vi "Frame1.vi"() -> ()   [LabVIEW 2017]
uses:
  <vilib>/myRIO/Instrument Drivers/Onboard IO/DIO/typedefs/DIO Reference.ctl
  <vilib>/myRIO/Common/Instrument Driver Framework/Utilities/typedefs/myRIO Generic Hardware Reference.ctl
  <vilib>/myRIO/Common/Instrument Driver Framework/Utilities/typedefs/Hardware Version Enum.ctl
  <vilib>/myRIO/Common/Instrument Driver Framework/Utilities/typedefs/myRIO v1.0 Reference.ctl
  <vilib>/myRIO/Common/Instrument Driver Framework/Utilities/typedefs/Generic FPGA Reference.ctl
  <vilib>/myRIO/Common/Instrument Driver Framework/myRIO v1.0/DIO/typedefs/DIO Channels List.ctl
  <vilib>/myRIO/Common/Instrument Driver Framework/myRIO v1.0/DIO/typedefs/DIO Channels Enum.ctl
  <vilib>/userdefined/High Color/nirio_resource_hc.ctl
  <vilib>/myRIO/Common/Instrument Driver Framework/Utilities/vis/Is FPGA Ref Available.vi
  <vilib>/myRIO/Common/Instrument Driver Framework/myRIO v1.0/DIO/vis/myRIO v1.1 Open DIO.vi
  <vilib>/myRIO/Instrument Drivers/Onboard IO/DIO/vis/Read.vi
  <vilib>/myRIO/Common/Instrument Driver Framework/Utilities/vis/Validate Channels.vi
  <vilib>/myRIO/Common/Instrument Driver Framework/myRIO v1.0/DIO/vis/myRIO v1.0 Reserve DIO.vi
  <vilib>/myRIO/Common/Instrument Driver Framework/myRIO v1.0/UART/vis/myRIO v1.0 Close UART.vi
  <vilib>/myRIO/Common/Instrument Driver Framework/myRIO v1.0/Resource Manager/vis/myRIO v1.0 Reserve Channel List.vi
  <vilib>/myRIO/Common/Instrument Driver Framework/myRIO v1.0/DIO/vis/myRIO v1.0 Build MUX Configuration DIO.vi
  <vilib>/myRIO/Common/Instrument Driver Framework/myRIO v1.0/Resource Manager/vis/myRIO v1.0 Reserve Channel.vi
  <vilib>/myRIO/Common/Instrument Driver Framework/myRIO v1.0/Resource Manager/vis/myRIO v1.0 Unreserve Channel.vi
  <vilib>/myRIO/Common/Instrument Driver Framework/myRIO v1.0/Resource Manager/vis/myRIO v1.0 Create Configuration List.vi
  <vilib>/myRIO/Common/Instrument Driver Framework/myRIO v1.0/Resource Manager/vis/myRIO v1.0 Build Mutex Name.vi
  <vilib>/Utility/VariantDataType/GetNumericInfo.vi
  <vilib>/Utility/error.llb/Error Cluster From Error Code.vi
  <vilib>/myRIO/Common/Instrument Driver Framework/myRIO v1.0/myRIO v1.1 Open.vi
  <vilib>/myRIO/Common/Instrument Driver Framework/Utilities/vis/IO Manager.vi
  <vilib>/myRIO/Common/Instrument Driver Framework/Utilities/vis/Configuration Manager.vi
  <vilib>/myRIO/Common/Instrument Driver Framework/myRIO v1.0/Resource Manager/vis/myRIO v1.0 Configure IO.vi
  <vilib>/myRIO/Common/Instrument Driver Framework/myRIO v1.0/myRIO v1.0 Close.vi
  <vilib>/myRIO/Common/Instrument Driver Framework/myRIO v1.0/DIO/vis/myRIO v1.0 Read DIO.vi
  <vilib>/myRIO/Common/Instrument Driver Framework/Utilities/vis/FPGA Ref Manager.vi
  <vilib>/myRIO/Common/Instrument Driver Framework/myRIO v1.0/myRIO v1.0 Reset FPGA.vi
  <vilib>/myRIO/Common/Instrument Driver Framework/myRIO v1.0/IRQ/vis/myRIO v1.0 IRQ Info FGV.vi
  <vilib>/myRIO/Common/Instrument Driver Framework/myRIO v1.0/IRQ/vis/myRIO v1.0 Timer IRQ Info FGV.vi
  <vilib>/myRIO/Common/Instrument Driver Framework/myRIO v1.0/IRQ/vis/myRIO v1.0 ISR Agent.vi
  <vilib>/myRIO/Express VI/Onboard Devices/Button/Button Express VI.xnode
  <vilib>/myRIO/Instrument Drivers/Onboard IO/DIO/vis/myRIO DIO Open.xnode
  <vilib>/myRIO/Instrument Drivers/Onboard IO/DIO/DIO.lvlib
  <vilib>/myRIO/Instrument Drivers/Utilities/Utilities.lvlib
panel:
  out "error out":errorcluster
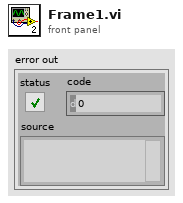
[diagram p1: front panel]
types:
  T1 = typedef "DIO.lvlib/DIO Reference.ctl" = cluster{"myRIO Reference":T2, "DIO Channels List":T6}
  T2 = typedef "myRIO Generic Hardware Reference.ctl" = cluster{"myRIO Model":T3, "myRIO Hardware Reference":T4}
  T3 = typedef "Hardware Version Enum.ctl" = enum16{"Unknown", "myRIO-1900", "myRIO-1950", "roboRIO", "NI ELVIS RIO CM"}
  T4 = typedef "myRIO v1.0 Reference.ctl" = cluster{"Generic FPGA Reference":T5, "Allow multiple opens":bool}
  T5 = typedef "Generic FPGA Reference.ctl" = refnum<k20>
  T6 = typedef "DIO Channels List.ctl" = T7[]
  T7 = typedef "DIO Channels Enum.ctl" = enum16{"Not Connected", "C/DIO0", "C/DIO1", "C/DIO2", "C/DIO3", "C/DIO4", "C/DIO5", "C/DIO6", "C/DIO7", "A/DIO0", "A/DIO1", "A/DIO2", "A/DIO3", "A/DIO4", "A/DIO5", "A/DIO6", "A/DIO7", "A/DIO8", "A/DIO9", "A/DIO10", "A/DIO11", "A/DIO12", "A/DIO13", "A/DIO14", "A/DIO15", "B/DIO0", "B/DIO1", "B/DIO2", "B/DIO3", "B/DIO4", "B/DIO5", "B/DIO6", "B/DIO7", "B/DIO8", "B/DIO9", "B/DIO10", "B/DIO11", "B/DIO12", "B/DIO13", "B/DIO14", "B/DIO15", "LED0", "LED1", "LED2", "LED3", "Button0", "DIO/DIO0", "DIO/DIO1", "DIO/DIO2", "DIO/DIO3", "DIO/DIO4", "DIO/DIO5", "DIO/DIO6", "DIO/DIO7", "DIO/DIO8", "DIO/DIO9", "SPI/CS0", "SPI/CS1", "SPI/CS2", "SPI/CS3", "LED RADIO (Green)", "LED RADIO (Red)", "LED COMM (Green)", "LED COMM (Red)", "LED MODE (Green)", "LED MODE (Red)"}
  T8 = typedef "nirio_resource_hc.ctl" = tag
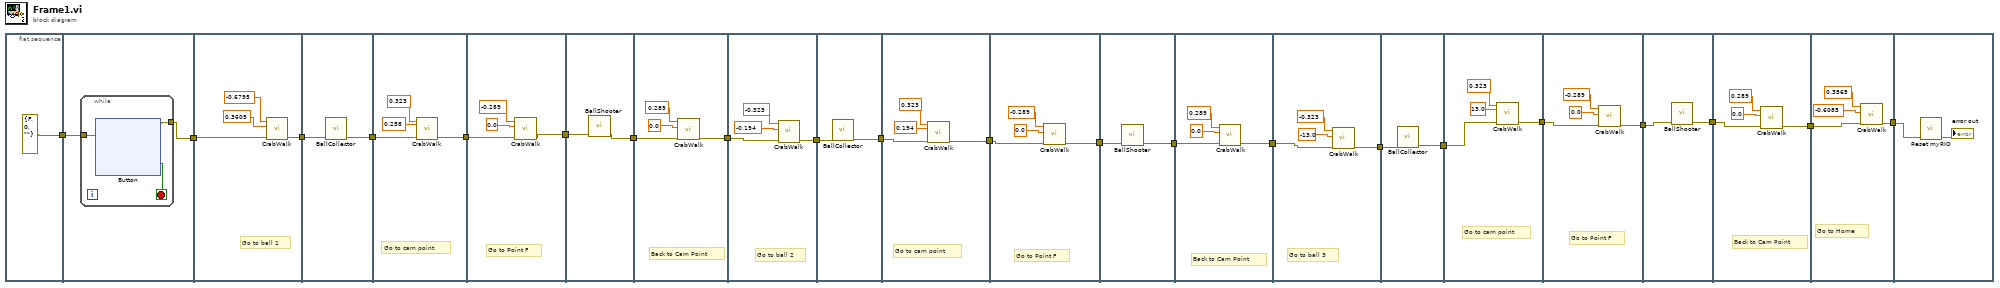
[diagram p0: block diagram]
diagram:
  n1 = flat-sequence {
    tunnel: [errorcluster {"status"=FALSE, "code"=0, "source"=""} ("error constant")] -> w21
    tunnel: w21 -> [w24]
    tunnel: [w23] -> w20
    tunnel: w20 -> [w66]
    tunnel: [w65] -> w19
    tunnel: w19 -> [w68]
    tunnel: [w67] -> w18
    tunnel: w18 -> [w72]
    tunnel: [w71] -> w17
    tunnel: w17 -> [w76]
    tunnel: [w73] -> w16
    tunnel: w16 -> [w78]
    tunnel: [w77] -> w15
    tunnel: w15 -> [w80]
    tunnel: [w79] -> w14
    tunnel: w14 -> [w84]
    tunnel: [w83] -> w13
    tunnel: w13 -> [w88]
    tunnel: [w87] -> w12
    tunnel: w12 -> [w90]
    tunnel: [w89] -> w11
    tunnel: w11 -> [w94]
    tunnel: [w93] -> w10
    tunnel: w10 -> [w98]
    tunnel: [w97] -> w9
    tunnel: w9 -> [w100]
    tunnel: [w99] -> w8
    tunnel: w8 -> [w104]
    tunnel: [w103] -> w7
    tunnel: w7 -> [w108]
    tunnel: [w107] -> w6
    tunnel: w6 -> [w110]
    tunnel: [w109] -> w5
    tunnel: w5 -> [w114]
    tunnel: [w113] -> w4
    tunnel: w4 -> [w118]
    tunnel: [w117] -> w3
    tunnel: w3 -> [w120]
    tunnel: [w119] -> w2
    tunnel: w2 -> [w124]
    tunnel: [w123] -> w1
    tunnel: w1 -> [w127]
    frame #0 {
    }
    frame #1 {
      n2 = while {
        tunnel: w24 -> [w27]
        tunnel: [w25] -> w23
        stop <- w26 stop-if-true
        n3 = xnode "Button"("error in (no error)"=w27) -> ("Value"=w26:bool, "error out"=w25:errorcluster)
      }
    }
    frame #2 {
      # "Go to ball 1"
      n4 = call "CrabWalk.vi"("error in\n(no error)"=w66, "Distance Y (m)"=0.3605, "Distance X (m)"=-0.6795) -> ("error out"=w65:errorcluster)  [unwired: 7 in, 1 out]
    }
    frame #3 {
      n5 = call "BallCollector.vi"("error in\n(no error)"=w68) -> ("error out"=w67:errorcluster)  [unwired: 10 in]
    }
    frame #4 {
      # "Go to cam point"
      n6 = call "CrabWalk.vi"("error in\n(no error)"=w72, "Distance Y (m)"=0.258, "Distance X (m)"=0.323) -> ("error out"=w71:errorcluster)  [unwired: 7 in, 1 out]
    }
    frame #5 {
      # "Go to Point F"
      n7 = call "CrabWalk.vi"("error in\n(no error)"=w76, "Distance Y (m)"=0.0, "Distance X (m)"=-0.289) -> ("error out"=w73:errorcluster)  [unwired: 7 in, 1 out]
    }
    frame #6 {
      n8 = call "BallShooter.vi"("error in (no error)"=w78) -> ("error out"=w77:errorcluster)  [unwired: 10 in]
    }
    frame #7 {
      # "Back to Cam Point"
      n9 = call "CrabWalk.vi"("error in\n(no error)"=w80, "Distance Y (m)"=0.0, "Distance X (m)"=0.289) -> ("error out"=w79:errorcluster)  [unwired: 7 in, 1 out]
    }
    frame #8 {
      # "Go to ball 2"
      n10 = call "CrabWalk.vi"("error in\n(no error)"=w84, "Distance Y (m)"=-0.194, "Distance X (m)"=-0.323) -> ("error out"=w83:errorcluster)  [unwired: 7 in, 1 out]
    }
    frame #9 {
      n11 = call "BallCollector.vi"("error in\n(no error)"=w88) -> ("error out"=w87:errorcluster)  [unwired: 10 in]
    }
    frame #10 {
      # "Go to cam point"
      n12 = call "CrabWalk.vi"("error in\n(no error)"=w90, "Distance Y (m)"=0.194, "Distance X (m)"=0.323) -> ("error out"=w89:errorcluster)  [unwired: 7 in, 1 out]
    }
    frame #11 {
      # "Go to Point F"
      n13 = call "CrabWalk.vi"("error in\n(no error)"=w94, "Distance Y (m)"=0.0, "Distance X (m)"=-0.289) -> ("error out"=w93:errorcluster)  [unwired: 7 in, 1 out]
    }
    frame #12 {
      n14 = call "BallShooter.vi"("error in (no error)"=w98) -> ("error out"=w97:errorcluster)  [unwired: 10 in]
    }
    frame #13 {
      # "Back to Cam Point"
      n15 = call "CrabWalk.vi"("error in\n(no error)"=w100, "Distance Y (m)"=0.0, "Distance X (m)"=0.289) -> ("error out"=w99:errorcluster)  [unwired: 7 in, 1 out]
    }
    frame #14 {
      # "Go to ball 3"
      n16 = call "CrabWalk.vi"("error in\n(no error)"=w104, "Distance Y (m)"=-13.0, "Distance X (m)"=-0.323) -> ("error out"=w103:errorcluster)  [unwired: 7 in, 1 out]
    }
    frame #15 {
      n17 = call "BallCollector.vi"("error in\n(no error)"=w108) -> ("error out"=w107:errorcluster)  [unwired: 10 in]
    }
    frame #16 {
      # "Go to cam point"
      n18 = call "CrabWalk.vi"("error in\n(no error)"=w110, "Distance Y (m)"=13.0, "Distance X (m)"=0.323) -> ("error out"=w109:errorcluster)  [unwired: 7 in, 1 out]
    }
    frame #17 {
      # "Go to Point F"
      n19 = call "CrabWalk.vi"("error in\n(no error)"=w114, "Distance Y (m)"=0.0, "Distance X (m)"=-0.289) -> ("error out"=w113:errorcluster)  [unwired: 7 in, 1 out]
    }
    frame #18 {
      n20 = call "BallShooter.vi"("error in (no error)"=w118) -> ("error out"=w117:errorcluster)  [unwired: 10 in]
    }
    frame #19 {
      # "Back to Cam Point"
      n21 = call "CrabWalk.vi"("error in\n(no error)"=w120, "Distance Y (m)"=0.0, "Distance X (m)"=0.289) -> ("error out"=w119:errorcluster)  [unwired: 7 in, 1 out]
    }
    frame #20 {
      # "Go to Home"
      n22 = call "CrabWalk.vi"("error in\n(no error)"=w124, "Distance Y (m)"=-0.6085, "Distance X (m)"=0.3565) -> ("error out"=w123:errorcluster)  [unwired: 7 in, 1 out]
    }
    frame #21 {
      n23 = call <vilib>:"Reset myRIO.vi"("error in (no error)"=w127) -> ("error out"=→"error out":errorcluster)  [unwired: 10 in]
    }
  }
